vi "Nastran PCH_Create.vi"(0 "reference in":refnum<class "Nastran PCH.lvclass">, 5 "error in (no error)":errorcluster, 7 "Application Name":string, 9 "State Queue":string[](array[string])) -> (14 "reference out":refnum<class "Nastran PCH.lvclass">, 19 "error out":errorcluster)   [LabVIEW 2022 SP3, in "Nastran PCH.lvclass"]
doc: "Constructor."
uses:
  Nastran PCH.lvclass
  C:/Program Files/National Instruments/LabVIEW 2022/vi.lib/addons/_AddQ/G#Object/G#Object.lvclass
  W:/projects/archives/23 Charette AI Group/SPWB/API/Generic Utilities_class/Generic Utilities.lvclass
  <vilib>/addons/_AddQ/G#Object/G#Object.lvclass
  API/Generic Utilities_class/Generic Utilities.lvclass
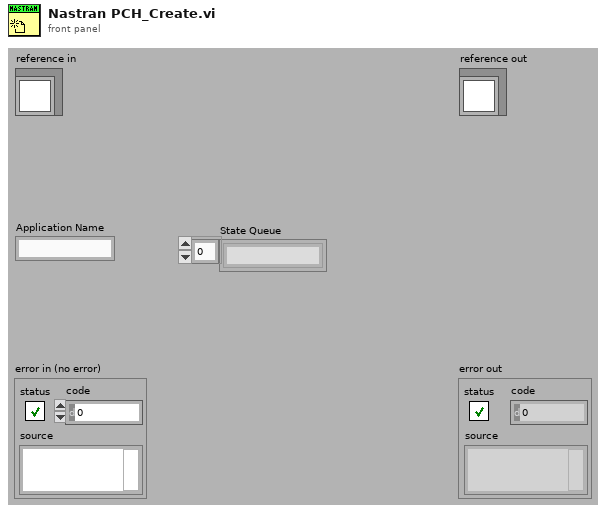
[diagram p1: front panel]
types:
  T1 = typedef "Nastran PCH.lvclass/ObjectAttributesRef.ctl" = refnum<data-value>
  T2 = typedef "Nastran PCH.lvclass/ObjectAttributes.ctl" = cluster{"FRF":cluster{"Title":string, "Sub Title":string, "Point ID":i32, "Subcase ID":i32, "Name":string, "Unit Type":enum16{"displacement", "velocity", "acceleration"}, "Unit":string, "Storage Type":enum16{"Sort1", "Sort2"}, "Abscissa":dbl[], "X":cdb[], "Y":cdb[], "Z":cdb[], "u":cdb[], "v":cdb[], "w":cdb[]}[]}
  T3 = cluster{"Title":string, "Sub Title":string, "Point ID":i32, "Subcase ID":i32, "Name":string, "Unit Type":enum16{"displacement", "velocity", "acceleration"}, "Unit":string, "Storage Type":enum16{"Sort1", "Sort2"}, "Abscissa":dbl[], "X":cdb[], "Y":cdb[], "Z":cdb[], "u":cdb[], "v":cdb[], "w":cdb[]}[]
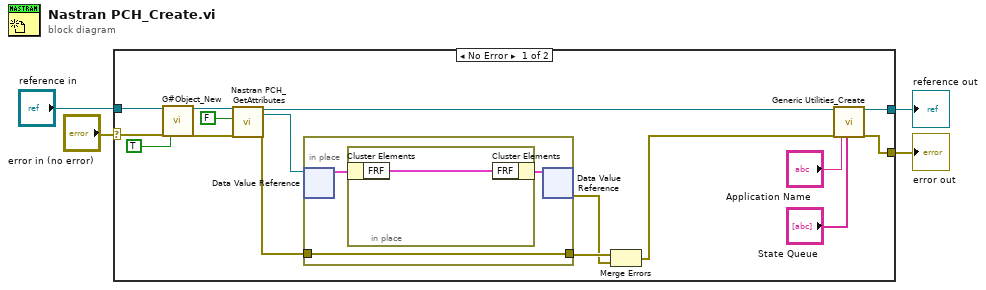
[diagram p0: block diagram]
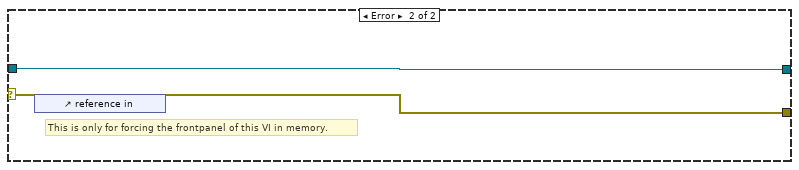
[diagram p2: hidden frame]
diagram:
  n1 = case shown="No Error" "error in (no error)" {
    selector: "error in (no error)" -> [w19 w26]
    tunnel: [w7 w26] -> w3
    tunnel: [w9 w25] -> w1
    tunnel: "reference in" -> [w20 w25]
    frame No Error {
      n2 = call <vilib>:"G#Object_New.vi"("reference in"=w20, "error in (no error)"=w19, "user counter (T)?"=TRUE ("User Counter")) -> ("reference out"=w12:refnum<class "Nastran PCH.lvclass">, "error out"=w11:errorcluster)  [unwired: 14 in, 1 out]
      n3 = call "Nastran PCH_GetAttributes.vi"("reference in"=w12, "return data? (T)"=FALSE ("return data"), "error in (no error)"=w11) -> ("reference out"=w10:refnum<class "Nastran PCH.lvclass">, "attributes ref"=w14:T1, "error out"=w15:errorcluster)  [unwired: 13 in, 1 out]
      n4 = in-place {
        in-place-border: w15 -> [w21]
        in-place-border: [w21] -> w17
        n5 = in-place-dvr #1(w14) -> (w22:T2)  [unwired: 1 out]
        n6 = in-place {
          n7 = in-place-cluster #2(w22) -> ("FRF"=w24:T3)
          n8 = in-place-cluster #2("FRF"=w24) -> (w23:T2)
        }
        n9 = in-place-dvr #1(w23) -> (w16:errorcluster)  [unwired: 1 out]
      }
      n10 = Merge Errors(w17, w16) -> (w8:errorcluster)
      n11 = call "Generic Utilities_Create.vi"("reference in"=w10, "error in (no error)"=w8, "Application Name"="Application Name", "State Queue"="State Queue") -> ("reference out"=w9:refnum<class "Nastran PCH.lvclass">, "error out"=w7:errorcluster)  [unwired: 14 in]
    }
    frame Error {
      # "This is only for forcing the frontpanel of this VI in memory."
      n12 = control-ref of="reference in"() -> ()  [unwired: 1 out]
    }
  }
  "error out" <- w3
  "reference out" <- w1
